vi "Insert Error.vi"(7 "scope":T2=enum."global", 8 "error in (no error)":errorcluster, 9 "new error":T1, 10 "owner path":string, 11 "error list <top> in":variant) -> (0 "error out":errorcluster, 3 "error list <top> out":variant)   [LabVIEW 2017]
uses:
  Scope.ctl
  Error File Management/Controls/NI Error.ctl
  Error File Management/Error File Management.lvlib
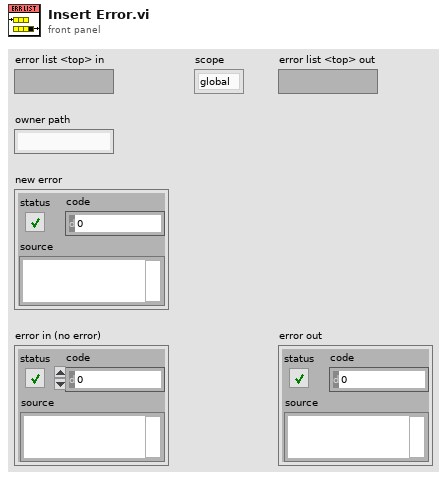
[diagram p1: front panel]
types:
  T1 = typedef "Error File Management.lvlib/NI Error.ctl" = errorcluster
  T2 = typedef "Scope.ctl" = enum16{"project", "global"}
  T3 = typedef "Error Code File Properties.ctl" = cluster{"path":path, "simplified path":string, "name":string, "display name":string, "family name":string, "comment":string, "parsable?":bool, "file modified?":bool}
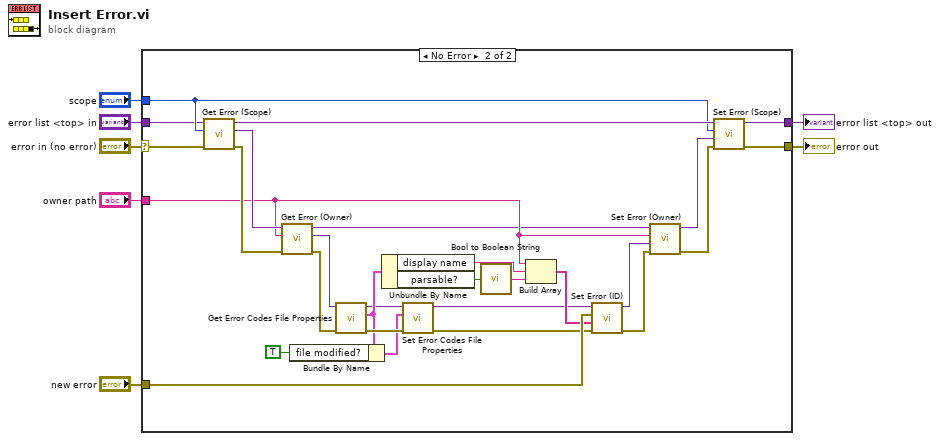
[diagram p0: block diagram]
diagram:
  n1 = case shown="No Error" "error in (no error)" {
    selector: "error in (no error)" -> [w9 w30]
    tunnel: "scope" -> [_ w32]
    tunnel: [w9 w31] -> w5
    tunnel: "error list <top> in" -> [w8 w29]
    tunnel: [w8 w28] -> w3
    tunnel: "new error" -> [_ w27]
    tunnel: "owner path" -> [_ w26]
    frame Error {
    }
    frame No Error {
      n2 = call "Get Error (Scope).vi"("error in (no error)"=w30, "scope"=w32, "error list <top>"=w29) -> ("error out"=w33:errorcluster, "error list <scope>"=w35:variant, "error list <top> dup"=w34:variant)  [unwired: 5 in, 1 out]
      n3 = call "Get Error (Owner).vi"("error in (no error)"=w33, "owner"=w26, "error list <scope>"=w35) -> ("error out"=w24:errorcluster, "error list <owner>"=w21:variant, "error list <scope> dup"=w25:variant)  [unwired: 5 in, 1 out]
      n4 = call "Get Error Codes File Properties.vi"("error in (no error)"=w24, "error list <owner> in"=w21) -> ("error out"=w22:errorcluster, "properties"=w15:T3, "error list <owner> out"=w12:variant)  [unwired: 6 in, 1 out]
      n5 = Bundle By Name(cluster=w15, "file modified?"=TRUE) -> (w10:T3)
      n6 = Unbundle By Name(w15) -> ("display name"=w19:string, "parsable?"=w20:bool)
      n7 = call "Set Error Codes File Properties.vi"("error in (no error)"=w22, "properties"=w10, "error list <owner> in"=w12) -> ("error out"=w13:errorcluster, "error list <owner> out"=w11:variant)  [unwired: 7 in]
      n8 = call "Bool to Boolean String.vi"("bool"=w20) -> ("boolean string"=w18:string)
      n9 = Build Array(w26, w19, w18) -> (w17:string[])
      n10 = call "Set Error (ID).vi"("error in (no error)"=w13, "attributes"=w17, "new error"=w27, "error list <owner> in"=w11) -> ("error out"=w23:errorcluster, "error list <owner> out"=w16:variant)  [unwired: 6 in]
      n11 = call "Set Error (Owner).vi"("error in (no error)"=w23, "error list <owner>"=w16, "owner"=w26, "error list <scope> in"=w25) -> ("error out"=w36:errorcluster, "error list <scope> out"=w37:variant)  [unwired: 6 in]
      n12 = call "Set Error (Scope).vi"("error in (no error)"=w36, "error list <scope>"=w37, "scope"=w32, "error list <top> in"=w34) -> ("error out"=w31:errorcluster, "error list <top> out"=w28:variant)  [unwired: 6 in]
    }
  }
  "error out" <- w5
  "error list <top> out" <- w3
